vi "TS_FILE_READER_frame.VI"(5 "error in (no error)":errorcluster, 6 "File":path) -> (0 "error out":errorcluster, 1 "S-parameter Array":cdb[][](array[numeric]) format="%.2f", 2 "Frequency Array":dbl[](array[numeric]) format="%.2e", 3 "Comments":string, 4 "Ref Impedance":u16=75)   [LabVIEW 2017]
doc: "Writes data in Freq S Real Imag or Magnitude Angle \n9 Column Touchstone format \nfeatures write protection for existing files"
panel:
  out "Data Format":enum16{"RI", "MA", "dB"}(ring)
  out "Freq Multiplier":dbl
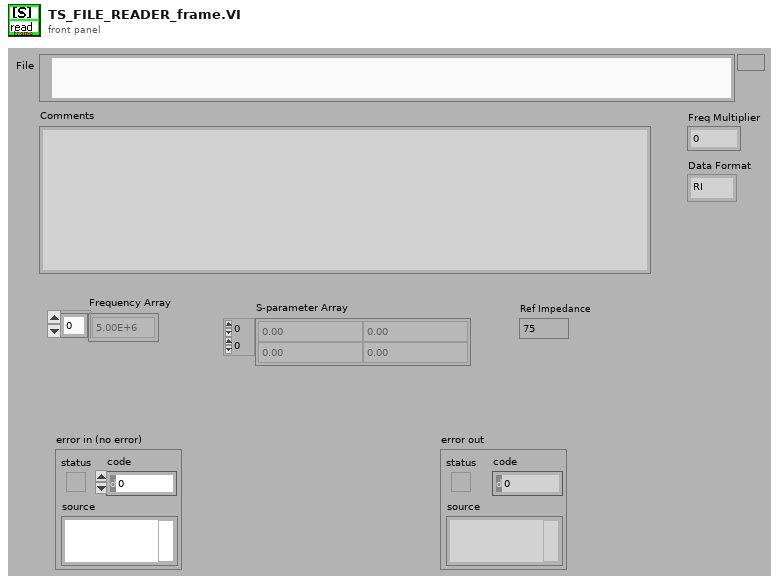
[diagram p1: front panel]
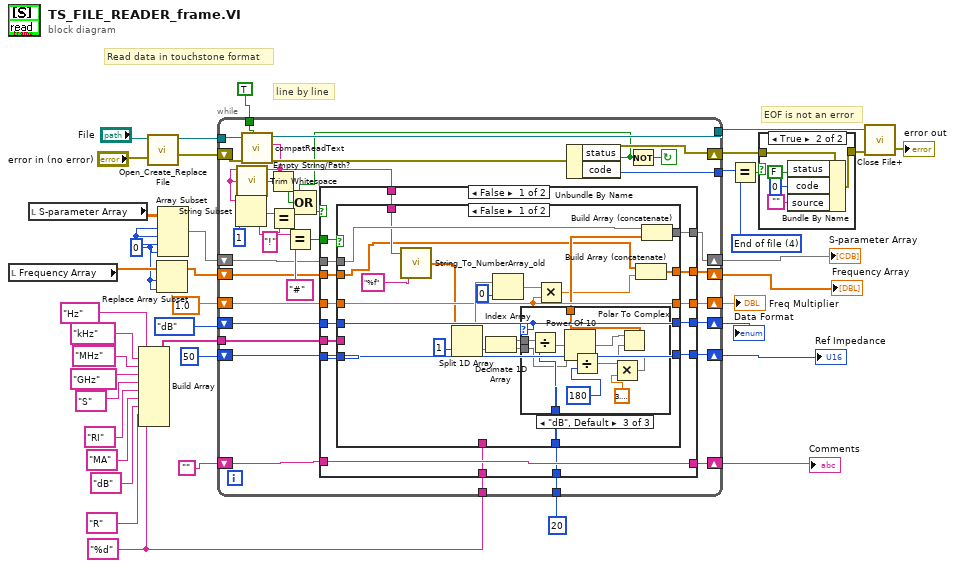
[diagram p0: block diagram]
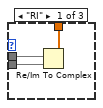
[diagram p3: hidden frame]
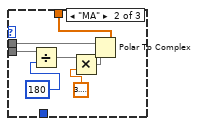
[diagram p4: hidden frame]
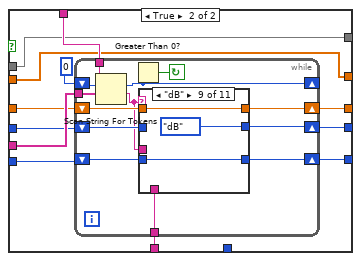
[diagram p5: hidden frame]
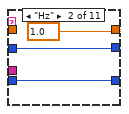
[diagram p7: hidden frame]
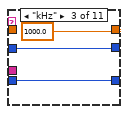
[diagram p8: hidden frame]
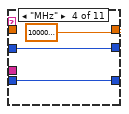
[diagram p9: hidden frame]
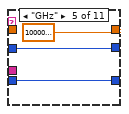
[diagram p10: hidden frame]
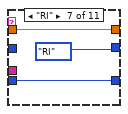
[diagram p12: hidden frame]
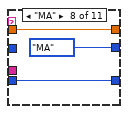
[diagram p13: hidden frame]
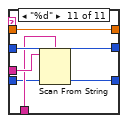
[diagram p15: hidden frame]
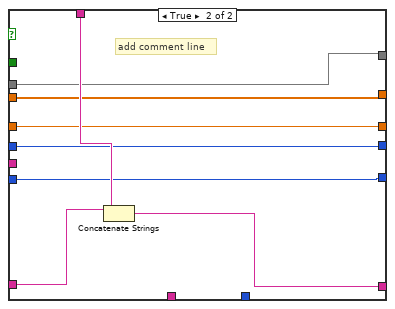
[diagram p16: hidden frame]
diagram:
  w3 = 0
  w19 = "%d"
  w32 = 4 items=["No error", "Argument error", "Memory is full", "Out of zone", "End of file", "File already open", "Generic file I/O error", "File not found", "File permission error", "Disk is full", "Duplicate path", "Too many files open", "System feature not enabled", "Resource file not found", "Cannot add resource", "Resource not found", "Image not found", "Image memory error", "Pen does not exist", "Config type invalid", "Config token not found", "Config parse error", "Config memory error", "Bad external code format", "Bad external code offset", "External code not present", "Null window", "Destroy window error", "Null menu", "Print aborted", "Bad print record", "Print driver error", "Windows error during printing", "Memory error during printing", "Print dialog error", "Generic print error", "Invalid device refnum", "Device not found", "Device parameter error", "Device unit error", "Cannot open device", "Device call aborted", "Generic error", "Cancelled by user", "Object ID too low", "Object ID too high", "Object not in heap", "Unknown heap", "Unknown object (invalid DefProc)", "Unknown object (DefProc not in table)", "Message out of range", "Invalid (null) method", "Unknown message", "Manager call not supported", "Bad address", "Network operation in progress", "Network operation timed out", "Connection is busy", "Network attribute not supported", "Network error", "Address in use", "System out of memory", "Connection aborted", "Connection refused", "Not connected", "Already connected", "Connection closed", "Initialization error (interapplication manager)", "Bad occurrence", "Wait on unbound occurrence handler", "Occurrence queue overflow", "Datalog type conflict", "Unused", "Unrecognized type (interapplication manager)", "Memory corrupt", "Failed to make temporary DLL", "Old CIN version", "Drag socket not found", "Failed to load drop-object", "Failed to register OLE object", "Failed to release OLE object", "Format specifier type mismatch", "Unknown format specifier", "Too few format specifiers", "Too many format specifiers", "Scan failed", "Newer CIN version", "Error converting to variant", "Runtime menu error", "Password tampered", "Variant attribute not found", "Incompatible variant data type", "Event data is not available", "Event Store is not present", "Occurrence is not found", "Event Queue is not created", "Event info is not available", "Refnum passed is NULL", "Error retrieving Class GUID", "Error retrieving CoClass GUID", "Error retrieving TypeLib GUID.", "Bad built application magic bytes.", "Specific driver is different from the specific driver associated with the Logical Name.", "There is no session opened to the class driver.", "Max Error", "MAX - Error with config objects", "MAX - Error loading configuration", "MAX - Group not supported"]
  # "line by line"
  # "EOF is not an error"
  # "Read data in touchstone format"
  n1 = local read "Frequency Array"() -> (w4:dbl[])
  n2 = local read "S-parameter Array"() -> (w8:cdb[][])
  n3 = Build Array("Hz", "kHz", "MHz", "GHz", "S", "RI", "MA", "dB", "R", w19) -> (w20:string[])
  n4 = call <vilib>:"Open_Create_Replace File.vi"("error in (no error)"="error in (no error)", "file path"="File") -> ("error out"=w36:errorcluster, "refnum"=w38:refnum<file>)  [unwired: 4 in, 4 out]
  n5 = Replace Array Subset(array=w4, new element=w3, index=w3) -> (w2:dbl[])
  n6 = Array Subset(array=w8, index (row)=w3, length (row)=w3, index (col)=w3, length (col)=w3) -> (w16:cdb[][])
  n7 = while {
    tunnel: [w70] -> w30
    tunnel: w38 -> [w72]
    tunnel: TRUE -> [w71]
    shift-right: [w68] -> w29
    shift-left: w36 -> [w69]
    tunnel: [w66] -> w33
    tunnel: w20 -> [w60]
    tunnel: w19 -> [w59]
    shift-right: [w56] -> w10
    shift-left: 1.0 -> [w57]
    shift-right: [w55] -> w6
    shift-left: u16 50 -> [w58]
    shift-right: [w53] -> w9
    shift-left: enum16{"RI", "MA", "dB"}."dB" -> [w54]
    shift-right: [w51] -> w7
    shift-left: w16 -> [w52]
    shift-right: [w49] -> w5
    shift-left: "" -> [w50]
    tunnel: 20 -> [w48]
    shift-right: [w40] -> w1
    shift-left: w2 -> [w41]
    stop <- w67 continue-if-true
    n8 = call <vilib>:"compatReadText.vi"("line mode (F)"=w71, "error in"=w69, "refnum"=w72) -> ("error out"=w68:errorcluster, "data"=w46:string, "dup refnum"=w70:refnum<file>)  [unwired: 2 in, 4 out]
    n9 = String Subset(string=w46, length (rest)=1) -> (substring=w64:string)  [unwired: 1 out]
    n10 = call <vilib>:"Trim Whitespace.vi"("string"=w46) -> ("trimmed string"=w47:string)  [unwired: 1 in]
    n11 = Empty String/Path?(string/path=w47) -> (empty?=w43:bool)
    n12 = Equal?(x=w64, y="!") -> (x = y?=w42:bool)
    n13 = Equal?(x=w64, y="#") -> (x = y?=w62:bool)
    n14 = Unbundle By Name(w68) -> ("status"=w44:bool, "code"=w66:i32)
    n15 = Compound Arithmetic op=OR(w44, w43, w42) -> (w45:bool)
    n16 = case shown="False" w45 {
      tunnel: w50 -> [w88 w196]
      tunnel: [w88 w195] -> w49
      tunnel: w46 -> [w86 w197]
      tunnel: w62 -> [w87 _]
      tunnel: w60 -> [w85 _]
      tunnel: w59 -> [w84 _]
      tunnel: [w83 w194] -> w55
      tunnel: w58 -> [w82 w194]
      tunnel: w57 -> [w81 w193]
      tunnel: [w80 w193] -> w56
      tunnel: w54 -> [w79 w192]
      tunnel: [w78 w192] -> w53
      tunnel: w52 -> [w77 w191]
      tunnel: [w76 w191] -> w51
      tunnel: w48 -> [w75 _]
      tunnel: w41 -> [w74 w190]
      tunnel: [w73 w190] -> w40
      frame False {
        n17 = case shown="False" w87 {
          tunnel: w86 -> [w95 w140]
          tunnel: w85 -> [_ w139]
          tunnel: w84 -> [_ w138]
          tunnel: [w108 w137] -> w83
          tunnel: w82 -> [w108 w136]
          tunnel: w81 -> [w97 w135]
          tunnel: [w97 w134] -> w80
          tunnel: w79 -> [w105 w132]
          tunnel: [w105 w131] -> w78
          tunnel: w77 -> [w102 w130]
          tunnel: [w99 w130] -> w76
          tunnel: w75 -> [w96 _]
          tunnel: w74 -> [w91 w129]
          tunnel: [w89 w129] -> w73
          frame False {
            n18 = call "String_To_NumberArray_old.vi"("Format"="%f", "Input String"=w95) -> ("Output Array"=w94:dbl[])
            n19 = Split 1D Array(array=w94, index=1) -> (first subarray=w101:dbl[], second subarray=w106:dbl[])
            n20 = Decimate 1D Array(w106) -> (w104:dbl[], w103:dbl[])
            n21 = Index Array(array=w101, index=0) -> (element=w98:dbl)
            n22 = case shown="\"dB\", Default" w105 {
              tunnel: w104 -> [w111 w118 w127]
              tunnel: w103 -> [w110 w116 w120]
              tunnel: [w109 w117 w128] -> w92
              tunnel: w96 -> [_ _ w126]
              frame "RI" {
                n23 = Re/Im To Complex(1:w110, 2:w111) -> (0:w109:cdb[])
              }
              frame "MA" {
                n24 = Divide(x=w116, y=180) -> (x/y=w114:dbl[])
                n25 = Multiply(x=w114, y=3.141592653589793) -> (x*y=w112:dbl[])
                n26 = Polar To Complex(1:w112, 2:w118) -> (0:w117:cdb[])
              }
              frame "dB", Default {
                n27 = Divide(x=w127, y=w126) -> (x/y=w125:dbl[])
                n28 = Power Of 10(x=w125) -> (10^x=w124:dbl[])
                n29 = Divide(x=w120, y=180) -> (x/y=w122:dbl[])
                n30 = Multiply(x=w122, y=3.141592653589793) -> (x*y=w119:dbl[])
                n31 = Polar To Complex(1:w119, 2:w124) -> (0:w128:cdb[])
              }
            }
            n32 = Multiply(x=w98, y=w97) -> (x*y=w90:dbl)
            n33 = Build Array (concatenate)(w91, w90) -> (w89:dbl[])
            n34 = Build Array (concatenate)(w102, w92) -> (w99:cdb[][])
          }
          frame True {
            n35 = while {
              shift-right: [w150] -> _
              shift-left: 0 -> [w152]
              tunnel: w140 -> [w153]
              tunnel: w139 -> [w149]
              shift-right: [w148] -> w134
              shift-left: w135 -> [w147]
              shift-right: [w146] -> w131
              shift-left: w132 -> [w145]
              tunnel: w138 -> [w144]
              shift-right: [w143] -> w137
              shift-left: w136 -> [w142]
              stop <- w151 continue-if-true
              n36 = Scan String For Tokens(7:w149, 8:w152, 9:w153) -> (1:w141:string, 2:w150:i32)  [unwired: 5 out]
              n37 = Greater Than 0?(x=w150) -> (x > 0?=w151:bool)
              n38 = case shown="\"dB\"" w141 {
                tunnel: [w156 1.0 1000.0 1000000.0 1000000000.0 w171 w174 w177 w180 w183 w189] -> w148
                tunnel: w147 -> [w156 _ _ _ _ w171 w174 w177 w180 w183 w189]
                tunnel: [w155 w158 w161 w164 w167 w170 enum16{"RI", "MA", "dB"}."RI" enum16{"RI", "MA", "dB"}."MA" enum16{"RI", "MA", "dB"}."dB" w182 w188] -> w146
                tunnel: w145 -> [w155 w158 w161 w164 w167 w170 _ _ _ w182 w188]
                tunnel: w141 -> [_ _ _ _ _ _ _ _ _ _ w187]
                tunnel: w144 -> [_ _ _ _ _ _ _ _ _ _ w186]
                tunnel: [w154 w157 w160 w163 w166 w169 w173 w176 w179 w181 w185] -> w143
                tunnel: w142 -> [w154 w157 w160 w163 w166 w169 w173 w176 w179 w181 w184]
                frame Default {
                }
                frame "Hz" {
                }
                frame "kHz" {
                }
                frame "MHz" {
                }
                frame "GHz" {
                }
                frame "S" {
                }
                frame "RI" {
                }
                frame "MA" {
                }
                frame "dB" {
                }
                frame "R" {
                }
                frame "%d" {
                  n39 = Scan From String(format string=w186, input string=w187, default 1=w184) -> (output 1=w185:u16)  [unwired: 2 in, 3 out]
                }
              }
            }
          }
        }
      }
      frame True {
        # "add comment line"
        n40 = Concatenate Strings(w196, w197) -> (w195:string)
      }
    }
    n41 = Not(x=w44) -> (.not. x?=w67:bool)
  }
  "Freq Multiplier" <- w10
  "Data Format" <- w9
  "Ref Impedance" <- w6
  "S-parameter Array" <- w7
  "Frequency Array" <- w1
  "Comments" <- w5
  n42 = Equal?(x=w33, y=w32) -> (x = y?=w31:bool)
  n43 = case shown="True" w31 {
    tunnel: w29 -> [w198 w203]
    tunnel: [w198 w199] -> w28
    frame False {
    }
    frame True {
      n44 = Bundle By Name(cluster=w203, "status"=FALSE, "code"=0, "source"="") -> (w199:errorcluster)
    }
  }
  n45 = call <vilib>:"Close File+.vi"("error in (no error)"=w28, "refnum"=w30) -> ("error out"=→"error out":errorcluster)  [unwired: 5 out]
